vi "Read Meta Data (Serial Ref).vi"(6 "options":T3={"ignore timeout error"=TRUE, "timeout ms (1000)"=1000}, 8 "error in":errorcluster, 11 "VISA resource name":refnum<visa-resource-name>) -> (0 "error out":errorcluster, 1 "meta data":T2[](array[typedef]), 3 "connection info out":T1)   [LabVIEW 2010, in "NI STM.lvlib"]
doc: "This VI reads the meta data information from a remote computer. Use this VI to retrieve the variable names and types that a remote computer exports.\n\nThis VI parses the data and returns a cluster containing the meta data information."
uses:
  NI STM.lvlib
  SubVIs/MetaDataElement.ctl
  Serial Read Options.ctl
  Serial Connection Info.ctl
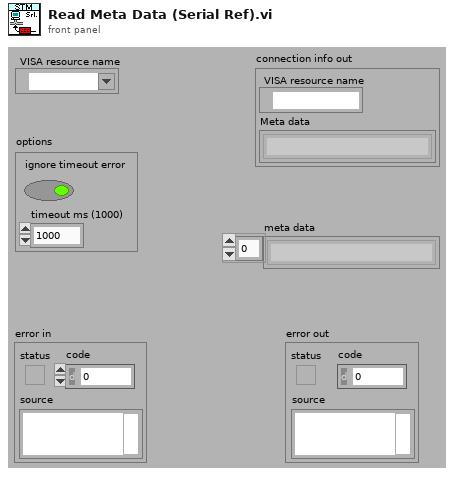
[diagram p1: front panel]
types:
  T1 = typedef "NI STM.lvlib/Serial Connection Info.ctl" = cluster{"VISA resource name":refnum<visa-resource-name>, "Meta data":T2[]}
  T2 = typedef "NI STM.lvlib/MetaDataElement.ctl" = string
  T3 = typedef "NI STM.lvlib/Serial Read Options.ctl" = cluster{"ignore timeout error":bool, "timeout ms (1000)":u32}
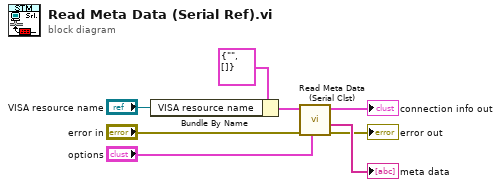
[diagram p0: block diagram]
diagram:
  n1 = Bundle By Name(cluster=T1 {"VISA resource name"="", "Meta data"=[]} ("Connection Info"), "VISA resource name"="VISA resource name") -> (w1:T1)
  n2 = call "Read Meta Data (Serial Clst).vi"("options"="options", "error in"="error in", "connection info in"=w1) -> ("error out"=→"error out":errorcluster, "meta data"=→"meta data":T2[], "connection info out"=→"connection info out":T1)  [unwired: 6 in]
